vi "CallEdge_CastToMoreSpecific.vi"(0 "reference":T1, 5 "error in (no error)":errorcluster) -> (14 "reference out":T1, 19 "error out":errorcluster)   [LabVIEW 2012, in "CallEdge.lvclass"]
doc: "CastToMoreSpecific"
uses:
  <resource>/Framework/Providers/Open_GDS/UML/CallEdge_class/CallEdge.lvclass
  <resource>/Framework/Providers/Open_GDS/UML/AbstractEdge_class/ObjectReference.ctl
  <vilib>/addons/_goop2.llb/GOOPStates.ctl
  <resource>/Framework/Providers/Open_GDS/UML/AbstractEdge_class/AbstractEdge.lvclass
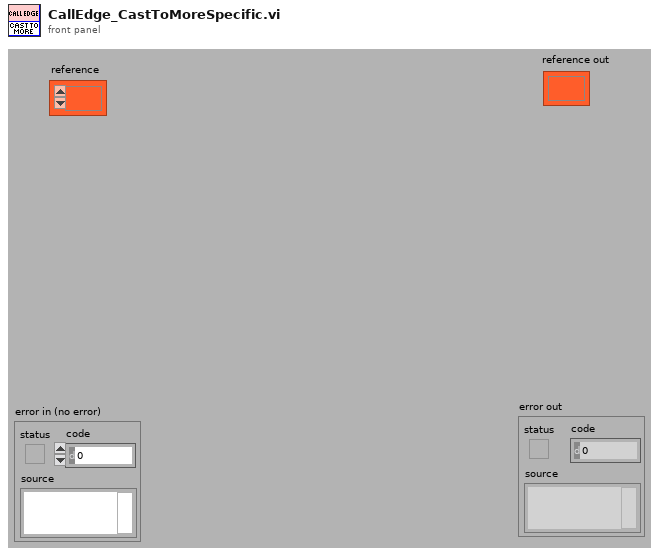
[diagram p1: front panel]
types:
  T1 = typedef "AbstractEdge.lvclass/ObjectReference.ctl" = refnum<k1>
  T2 = typedef "GOOPStates.ctl" = enum16{"Set", "Get", "New", "Delete", "Clear", "Test and get", "Unlock data", "Information", "Look up existing", "New or look up existing", "Test and get shared", "Get shared", "Set shared", "Unlock shared", "Find dynamic method", "Register dynamic method", "Preload dynamic method", "Probe", "Cast to more generic", "Cast to more specific"}
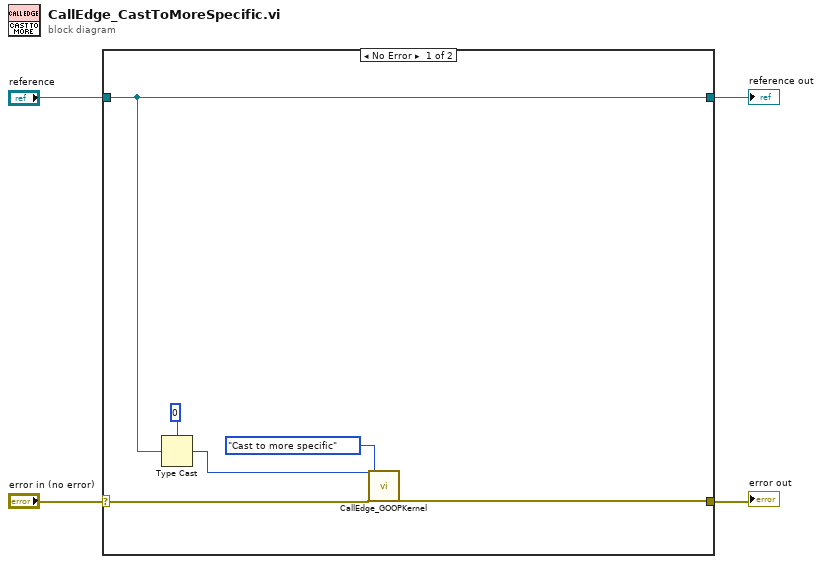
[diagram p0: block diagram]
diagram:
  n1 = case shown="No Error" "error in (no error)" {
    selector: "error in (no error)" -> [w7 w12]
    tunnel: [w6 w12] -> w3
    tunnel: "reference" -> [w5 w11]
    tunnel: [w5 w11] -> w2
    frame No Error {
      n2 = Type Cast(type=0, x=w5) -> (*(type *) &x=w8:i32)
      n3 = call <resource>:"CallEdge_GOOPKernel.vi"("Ref in"=w8, "error in (no error)"=w7, "Action"=GOOPStates."Cast to more specific") -> ("error out"=w6:errorcluster)  [unwired: 12 in, 12 out]
    }
    frame Error {
    }
  }
  "error out" <- w3
  "reference out" <- w2
